vi "OldIntakeStateMachine.vi"(8 "error in (no error)":errorcluster, 9 "IntakeCancel":bool, 10 "IntakeCommand":bool[](array[boolean]), 11 "Sensor_HaveNote":bool) -> (0 "error out":errorcluster, 1 "Intake_State":T1, 2 "MotorOutDmd 2":dbl, 3 "MotorOutDmd":dbl)   [LabVIEW 2023]
doc: "Process Intake State Machine"
uses:
  OldIntakeState.ctl
  OldIntakeGlobal.vi
panel:
  # "Click here to set min"
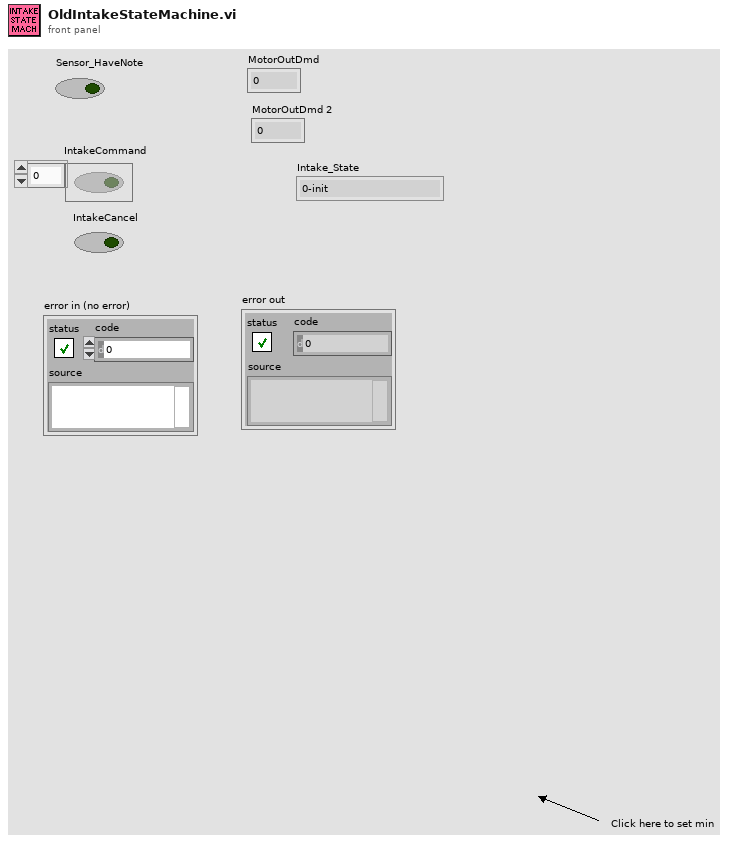
[diagram p1: front panel]
types:
  T1 = typedef "OldIntakeState.ctl" = enum16{"0-init", "1-cancel", "2-wait-for-cmd", "3-intake-check-for-note", "4-intake-start-intake", "5-intake-have-note-yet", "6-intake-stop-motor", "7-spit-out", "8-feed-note-to-shooter"}
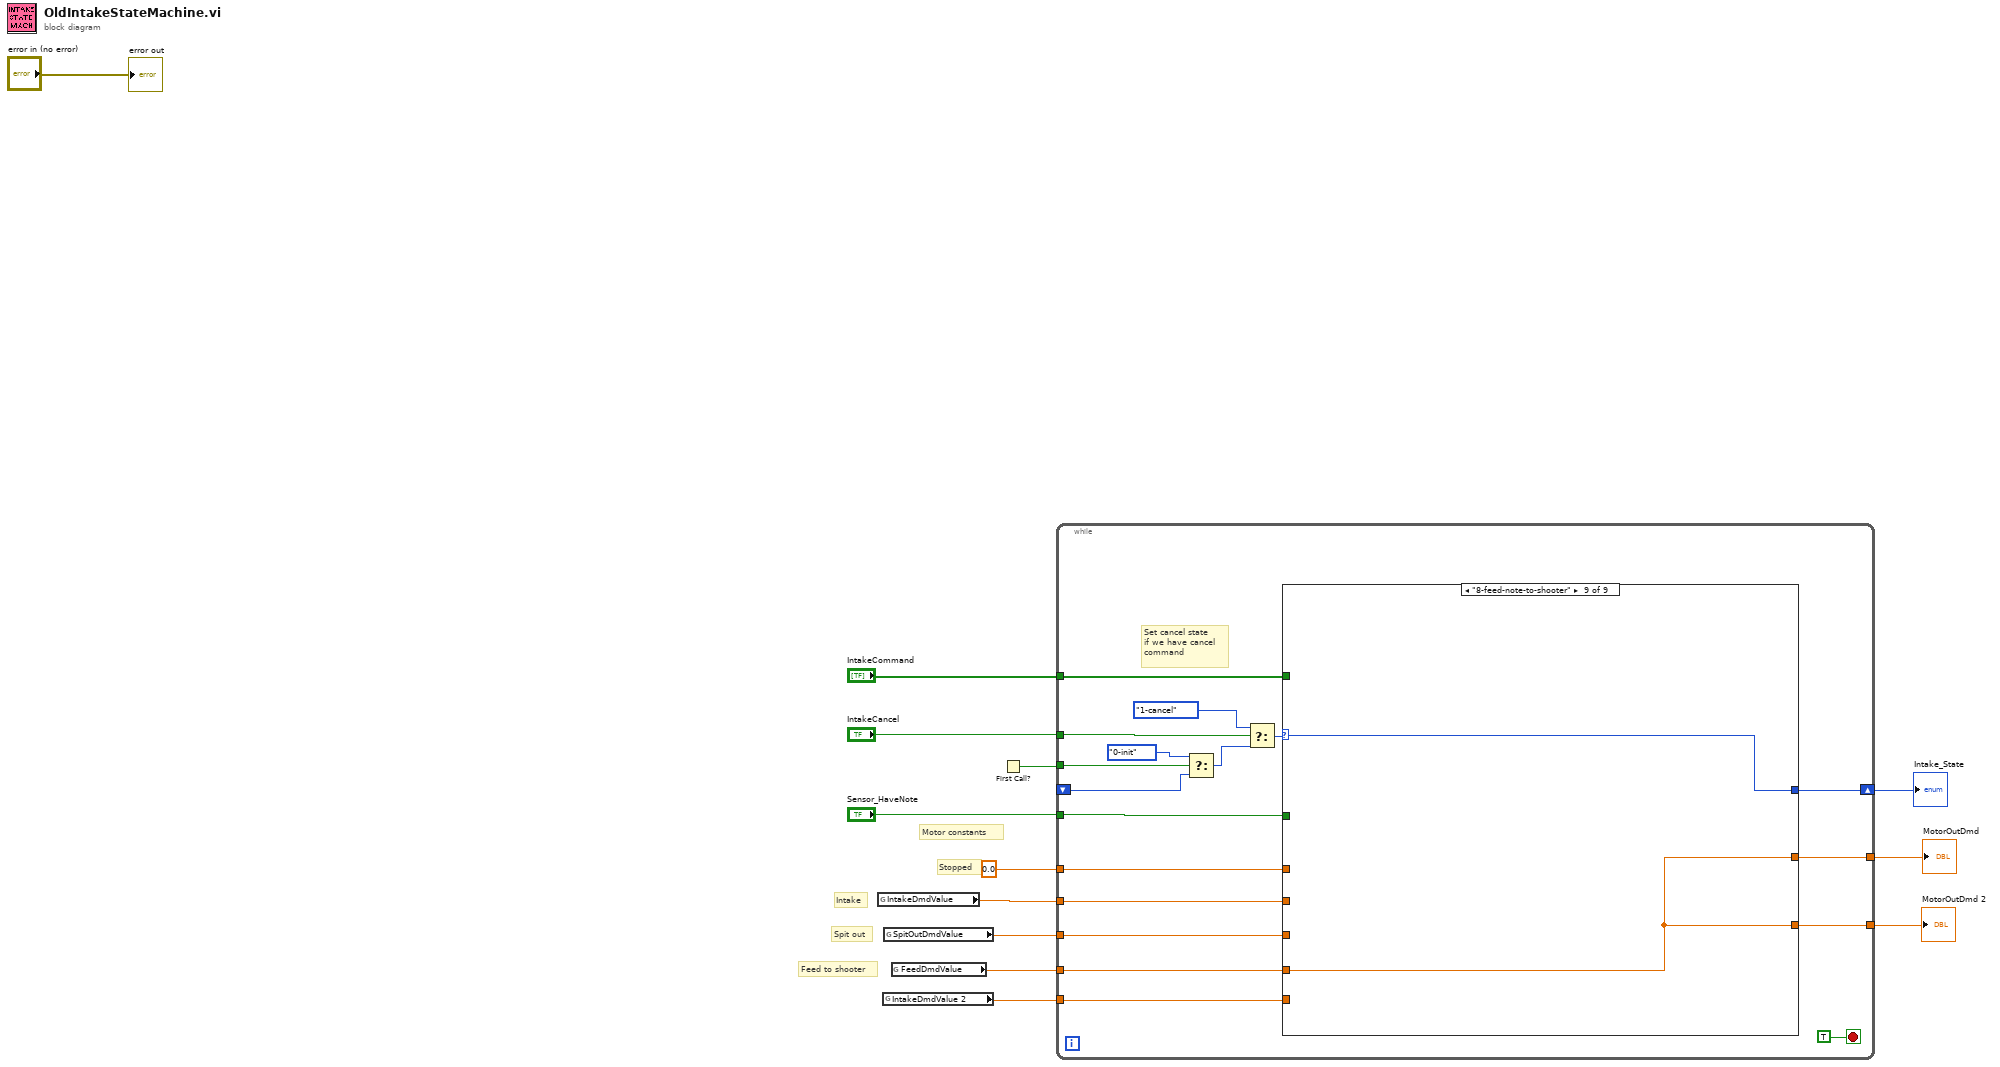
[diagram p0: block diagram]
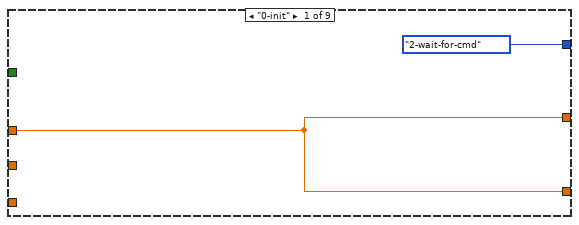
[diagram p2: hidden frame]
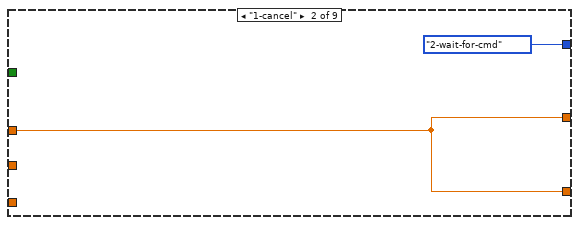
[diagram p3: hidden frame]
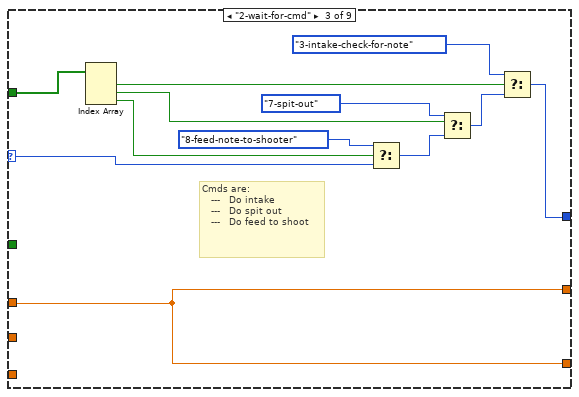
[diagram p4: hidden frame]
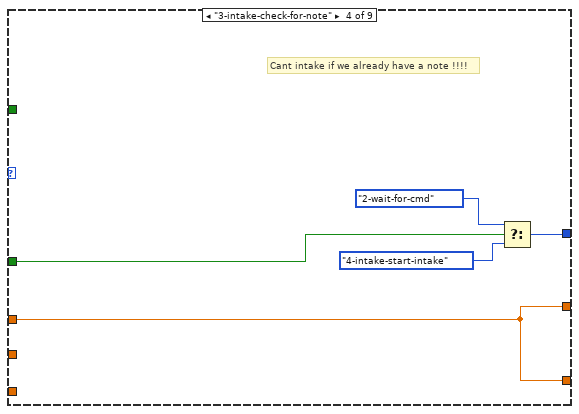
[diagram p5: hidden frame]
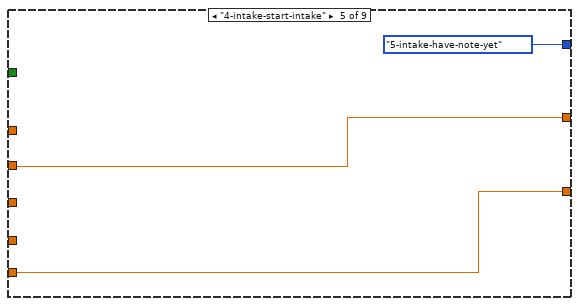
[diagram p6: hidden frame]
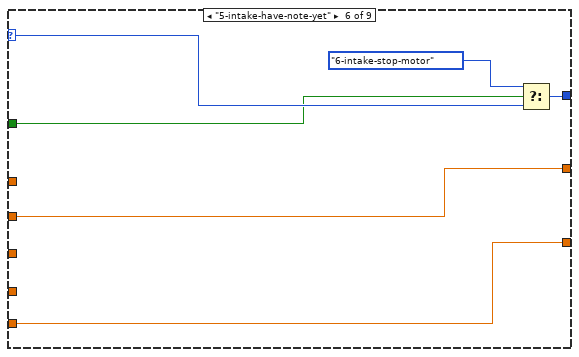
[diagram p7: hidden frame]
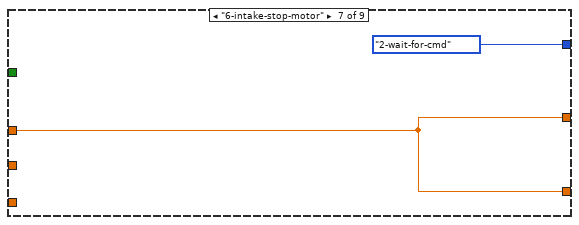
[diagram p8: hidden frame]
diagram:
  # "Feed to shooter"
  # "Spit out"
  # "Intake"
  # "Stopped"
  # "Motor constants"
  n1 = global read "OldIntakeGlobal.vi" "IntakeDmdValue"() -> (w5:dbl)
  n2 = global read "OldIntakeGlobal.vi" "IntakeDmdValue 2"() -> (w2:dbl)
  n3 = global read "OldIntakeGlobal.vi" "SpitOutDmdValue"() -> (w3:dbl)
  n4 = global read "OldIntakeGlobal.vi" "FeedDmdValue"() -> (w4:dbl)
  n5 = First Call?() -> (First Call?: T/F=w8:bool)
  n6 = while {
    tunnel: "IntakeCommand" -> [w31]
    tunnel: "Sensor_HaveNote" -> [w30]
    tunnel: [w29] -> w10
    tunnel: "IntakeCancel" -> [w23]
    shift-right: [w25] -> w6
    shift-left: _ -> [w20]
    tunnel: w8 -> [w21]
    tunnel: w4 -> [w19]
    tunnel: w3 -> [w18]
    tunnel: w5 -> [w17]
    tunnel: 0.0 -> [w16]
    tunnel: w2 -> [w15]
    tunnel: [w14] -> w1
    stop <- TRUE stop-if-true
    # "Set cancel state\nif we have cancel\ncommand"
    n7 = Select(t=OldIntakeState."0-init" ("Box Note State"), s=w21, f=w20) -> (s? t:f=w22:T1)
    n8 = Select(t=OldIntakeState."1-cancel" ("Box Note State"), s=w23, f=w22) -> (s? t:f=w27:T1)
    n9 = case shown="\"8-feed-note-to-shooter\"" w27 {
      selector: w27 -> [_ _ w39 _ _ w60 _ w65 w67]
      tunnel: [w32 w34 w36 w48 w54 w61 w62 w64 w66] -> w29
      tunnel: w31 -> [_ _ w47 _ _ _ _ _ _]
      tunnel: w30 -> [_ _ _ w52 _ w59 _ _ _]
      tunnel: w17 -> [_ _ _ _ w54 w61 _ _ _]
      tunnel: w16 -> [w32 w34 w36 w48 _ _ w62 _ _]
      tunnel: w18 -> [_ _ _ _ _ _ _ w64 _]
      tunnel: w19 -> [_ _ _ _ _ _ _ _ w66]
      tunnel: [OldIntakeState."2-wait-for-cmd" ("Box Note State") OldIntakeState."2-wait-for-cmd" ("Box Note State") w37 w50 OldIntakeState."5-intake-have-note-yet" ("Box Note State") w57 OldIntakeState."2-wait-for-cmd" ("Box Note State") w65 w67] -> w25
      tunnel: w15 -> [_ _ _ _ w53 w56 _ _ _]
      tunnel: [w32 w34 w36 w48 w53 w56 w62 w64 w66] -> w14
      frame "0-init" {
      }
      frame "1-cancel" {
      }
      frame "2-wait-for-cmd" {
        # "Cmds are:\n   ---   Do intake\n   ---   Do spit out\n   ---   Do feed to shoot"
        n10 = Index Array(array=w47) -> (element #1=w43:bool, element #2=w45:bool, element #3=w44:bool)  [unwired: 3 in]
        n11 = Select(t=OldIntakeState."8-feed-note-to-shooter" ("Box Note State"), s=w44, f=w39) -> (s? t:f=w46:T1)
        n12 = Select(t=OldIntakeState."7-spit-out" ("Box Note State"), s=w45, f=w46) -> (s? t:f=w38:T1)
        n13 = Select(t=OldIntakeState."3-intake-check-for-note" ("Box Note State"), s=w43, f=w38) -> (s? t:f=w37:T1)
      }
      frame "3-intake-check-for-note" {
        # "Cant intake if we already have a note !!!!"
        n14 = Select(t=OldIntakeState."2-wait-for-cmd" ("Box Note State"), s=w52, f=OldIntakeState."4-intake-start-intake" ("Box Note State")) -> (s? t:f=w50:T1)
      }
      frame "4-intake-start-intake" {
      }
      frame "5-intake-have-note-yet" {
        n15 = Select(t=OldIntakeState."6-intake-stop-motor" ("Box Note State"), s=w59, f=w60) -> (s? t:f=w57:T1)
      }
      frame "6-intake-stop-motor" {
      }
      frame "7-spit-out" {
      }
      frame "8-feed-note-to-shooter" {
      }
    }
  }
  "MotorOutDmd" <- w10
  "Intake_State" <- w6
  "MotorOutDmd 2" <- w1
  "error out" <- "error in (no error)"
